vi "Is Target.vi"() -> ()   [LabVIEW 2018, in "Tests.lvlib" / "Toolkit.lvlib" / "Integration.lvlib"]
uses:
  Integration.lvlib
panel:
  in  "Input 2":bool[](array[boolean])=[FALSE, FALSE, FALSE, TRUE, FALSE, FALSE]
  out "Any? 2":bool
  in  "Input":bool[](array[boolean])=[FALSE, FALSE, FALSE, TRUE, FALSE, FALSE]
  out "Any?":bool
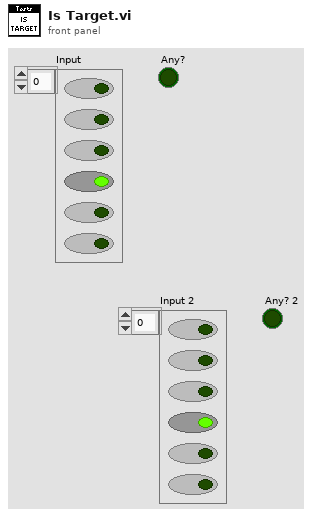
[diagram p1: front panel]
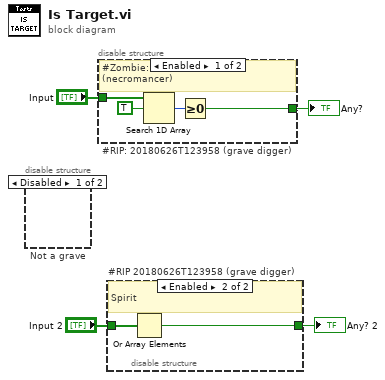
[diagram p0: block diagram]
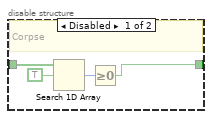
[diagram p2: hidden frame]
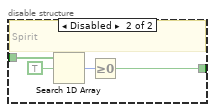
[diagram p4: hidden frame]
diagram:
  n1 = disable-structure "Not a grave" shown="Disabled" {
    frame Disabled {
    }
    frame Enabled {
    }
  }
  n2 = disable-structure "#RIP: 20180626T123958 (grave digger)" shown="Enabled" {
    disable-tunnel: "Input" -> [w8 w12]
    disable-tunnel: [w7 w11] -> w3
    frame Enabled {
      # "#Zombie: 20180626T124155 (necromancer)"
      n3 = Search 1D Array(1D array=w8, element=TRUE) -> (index of element=w5:i32)  [unwired: 1 in]
      n4 = Greater Or Equal To 0?(x=w5) -> (x >= 0?=w7:bool)
    }
    frame Disabled {
      # "Spirit"
      n5 = Search 1D Array(1D array=w12, element=TRUE) -> (index of element=w9:i32)  [unwired: 1 in]
      n6 = Greater Or Equal To 0?(x=w9) -> (x >= 0?=w11:bool)
    }
  }
  "Any?" <- w3
  n7 = disable-structure "#RIP 20180626T123958 (grave digger)" shown="Enabled" {
    disable-tunnel: "Input 2" -> [w16 w18]
    disable-tunnel: [w15 w17] -> w1
    frame Disabled {
      # "Corpse"
      n8 = Search 1D Array(1D array=w16, element=TRUE) -> (index of element=w13:i32)  [unwired: 1 in]
      n9 = Greater Or Equal To 0?(x=w13) -> (x >= 0?=w15:bool)
    }
    frame Enabled {
      # "Spirit"
      n10 = Or Array Elements(Boolean array=w18) -> (logical OR=w17:bool)
    }
  }
  "Any? 2" <- w1
